vi "AlliGator Compute Lifetime Simulation Histograms.vi"(0 "tau 1":dbl[](array[numeric]), 5 "tau 2":dbl[](array[numeric]), 7 "a1":dbl[](array[numeric]), 9 "Histogram Options":T1={"Histogram Bin Size (Lifetime)"=1.0000000000000002e-10, "Histogram Bin Size (a1)"=0.1, "Histogram Upper Percentile"=100.0, "Histogram Lower Percentile"=0.0, "Histogram Fit"=FALSE}, 11 "Error In":errorcluster) -> (3 "Histograms":cluster{"Axis":dbl[], "Histogram":dbl[]}[](array[cluster]), 4 "Array Statistic (tau 1)":T2, 6 "Array Statistics (tau 2)":T2, 8 "Array Statistics (a1)":T2, 10 "Array of Scales":cluster{"X Scale":u32, "Y Scale":u32}[](array[cluster]), 13 "Plot Names":string[](array[string]), 14 "Message":string, 15 "Error Out":errorcluster)   [LabVIEW 2021, in "AlliGator Fit Method Benchmark.lvlib"]
doc: "Computes fitted parameter histograms and statistics."
uses:
  AlliGator Fit Method Benchmark.lvlib
  Arrays/Array Statistics.ctl
  AlliGator FMB Histogram Options.ctl
  Histograms/Linear Histogram Options.ctl
  Histograms/Histogram Bin Option.ctl
  Histograms/Histogram Bin Position.ctl
  5e0c3266-499e-46b2-80ef-c194e49f915b.vi
  9765538f-b151-4b8e-9b71-29b00fbc2fe4.vi
  8faa86fc-1a47-49e1-a18e-559db2184d30.vi
  c2a6bf4c-2b36-4ed5-885f-cf0e0406484b.vi
  6ac06ea2-d37e-43e0-baed-35fadc42c3ab.vi
  6045f332-e983-43bb-9ace-d0f5cff48457.vi
  dfa1e9a8-16d4-484e-b1d6-6a58a8855e91.vi
  5e0c3266-499e-46b2-80ef-c194e49f915b.vi/1ce800e1-bcd7-4855-83e2-66cab3687e54.vi
  9765538f-b151-4b8e-9b71-29b00fbc2fe4.vi/1ce800e1-bcd7-4855-83e2-66cab3687e54.vi
  8faa86fc-1a47-49e1-a18e-559db2184d30.vi/1ce800e1-bcd7-4855-83e2-66cab3687e54.vi
  c2a6bf4c-2b36-4ed5-885f-cf0e0406484b.vi/b1828c6e-eb0a-43e9-a724-8b596c52e435.vi
  c2a6bf4c-2b36-4ed5-885f-cf0e0406484b.vi/7a6138ed-c001-4311-b538-9ba42ae7c7b1.vi
  c2a6bf4c-2b36-4ed5-885f-cf0e0406484b.vi/52c6b4fa-501b-4af0-803b-8bab516ca5d3.vi
  c2a6bf4c-2b36-4ed5-885f-cf0e0406484b.vi/d7237e10-35ab-4bcb-a0c6-4883c3f4c990.vi
  c2a6bf4c-2b36-4ed5-885f-cf0e0406484b.vi/5fb5dd96-3b97-4592-ba56-58181c8e7105.vi
  c2a6bf4c-2b36-4ed5-885f-cf0e0406484b.vi/8e13a849-a393-4484-9968-4af7b25c38d7.vi
  6ac06ea2-d37e-43e0-baed-35fadc42c3ab.vi/b1828c6e-eb0a-43e9-a724-8b596c52e435.vi
  6ac06ea2-d37e-43e0-baed-35fadc42c3ab.vi/7a6138ed-c001-4311-b538-9ba42ae7c7b1.vi
  6ac06ea2-d37e-43e0-baed-35fadc42c3ab.vi/52c6b4fa-501b-4af0-803b-8bab516ca5d3.vi
  6ac06ea2-d37e-43e0-baed-35fadc42c3ab.vi/d7237e10-35ab-4bcb-a0c6-4883c3f4c990.vi
  6ac06ea2-d37e-43e0-baed-35fadc42c3ab.vi/5fb5dd96-3b97-4592-ba56-58181c8e7105.vi
  6ac06ea2-d37e-43e0-baed-35fadc42c3ab.vi/8e13a849-a393-4484-9968-4af7b25c38d7.vi
  6045f332-e983-43bb-9ace-d0f5cff48457.vi/b1828c6e-eb0a-43e9-a724-8b596c52e435.vi
  6045f332-e983-43bb-9ace-d0f5cff48457.vi/7a6138ed-c001-4311-b538-9ba42ae7c7b1.vi
  6045f332-e983-43bb-9ace-d0f5cff48457.vi/52c6b4fa-501b-4af0-803b-8bab516ca5d3.vi
  6045f332-e983-43bb-9ace-d0f5cff48457.vi/d7237e10-35ab-4bcb-a0c6-4883c3f4c990.vi
  6045f332-e983-43bb-9ace-d0f5cff48457.vi/5fb5dd96-3b97-4592-ba56-58181c8e7105.vi
  6045f332-e983-43bb-9ace-d0f5cff48457.vi/8e13a849-a393-4484-9968-4af7b25c38d7.vi
  dfa1e9a8-16d4-484e-b1d6-6a58a8855e91.vi/b1828c6e-eb0a-43e9-a724-8b596c52e435.vi
  dfa1e9a8-16d4-484e-b1d6-6a58a8855e91.vi/7a6138ed-c001-4311-b538-9ba42ae7c7b1.vi
  dfa1e9a8-16d4-484e-b1d6-6a58a8855e91.vi/52c6b4fa-501b-4af0-803b-8bab516ca5d3.vi
  dfa1e9a8-16d4-484e-b1d6-6a58a8855e91.vi/d7237e10-35ab-4bcb-a0c6-4883c3f4c990.vi
  dfa1e9a8-16d4-484e-b1d6-6a58a8855e91.vi/5fb5dd96-3b97-4592-ba56-58181c8e7105.vi
  dfa1e9a8-16d4-484e-b1d6-6a58a8855e91.vi/8e13a849-a393-4484-9968-4af7b25c38d7.vi
  Time/High Resolution Timing.vi
  <userlib>/_OpenG.lib/array/array.llb/Filter 1D Array__ogtk.vi
  <userlib>/_OpenG.lib/array/array.llb/Filter 1D Array (DBL)__ogtk.vi
  <userlib>/_OpenG.lib/array/array.llb/Delete Elements from Array__ogtk.vi
  <userlib>/_OpenG.lib/array/array.llb/Delete Elements from 1D Array (DBL)__ogtk.vi
  <vilib>/Utility/error.llb/Error Cluster From Error Code.vi
  Histograms/Histogram Window.lvlib
  Arrays/Arrays.lvlib
  Variant/Variant.lvlib
panel:
  # "see the AlliGator License on the block diagram (Ctrl+E or Window:Show Block Diagram)"
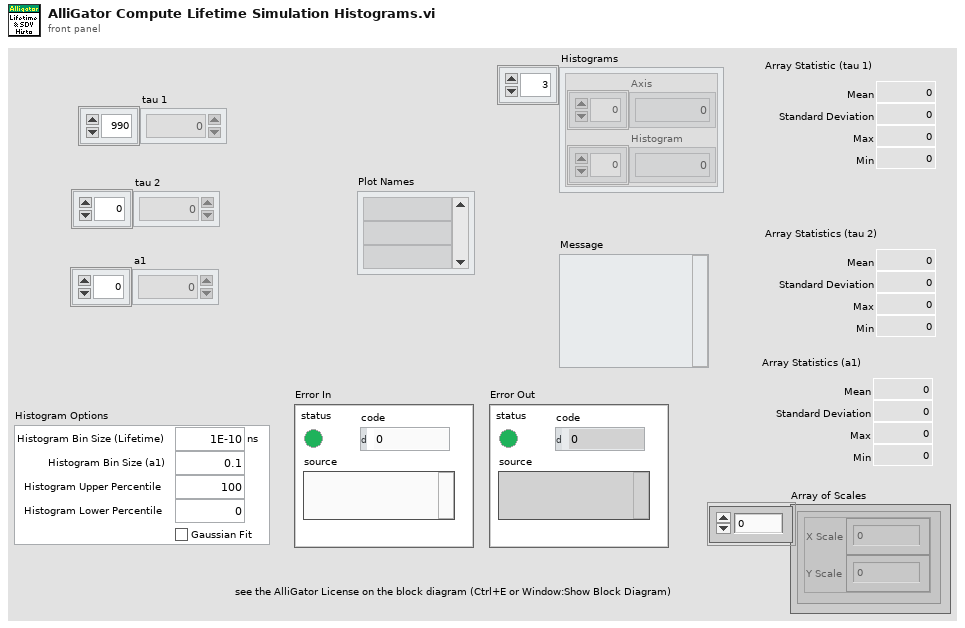
[diagram p1: front panel]
types:
  T1 = typedef "AlliGator Fit Method Benchmark.lvlib/AlliGator FMB Histogram Options.ctl" = cluster{"Histogram Bin Size (Lifetime)":dbl[unit], "Histogram Bin Size (a1)":dbl, "Histogram Upper Percentile":dbl, "Histogram Lower Percentile":dbl, "Histogram Fit":bool}
  T2 = typedef "Arrays.lvlib/Array Statistics.ctl" = cluster{"Mean":dbl, "Standard Deviation":dbl, "Max":dbl, "Min":dbl}
  T3 = typedef "Histogram Window.lvlib/Linear Histogram Options.ctl" = cluster{"Bin Size":dbl, "Bin Number":i32, "Bin Option":T4, "Min Value":dbl, "Max Value":dbl, "Filter NaN & Infinite Values":bool, "Frequency Plot":bool, "Align Bins":bool, "Bin Location":T5, "Project Outside Values":bool, "Max Histogram Size":i32}
  T4 = typedef "Histogram Window.lvlib/Histogram Bin Option.ctl" = enum32{"Bin Number", "Bin Size"}
  T5 = typedef "Histogram Window.lvlib/Histogram Bin Position.ctl" = enum16{"Left", "Center", "Right"}
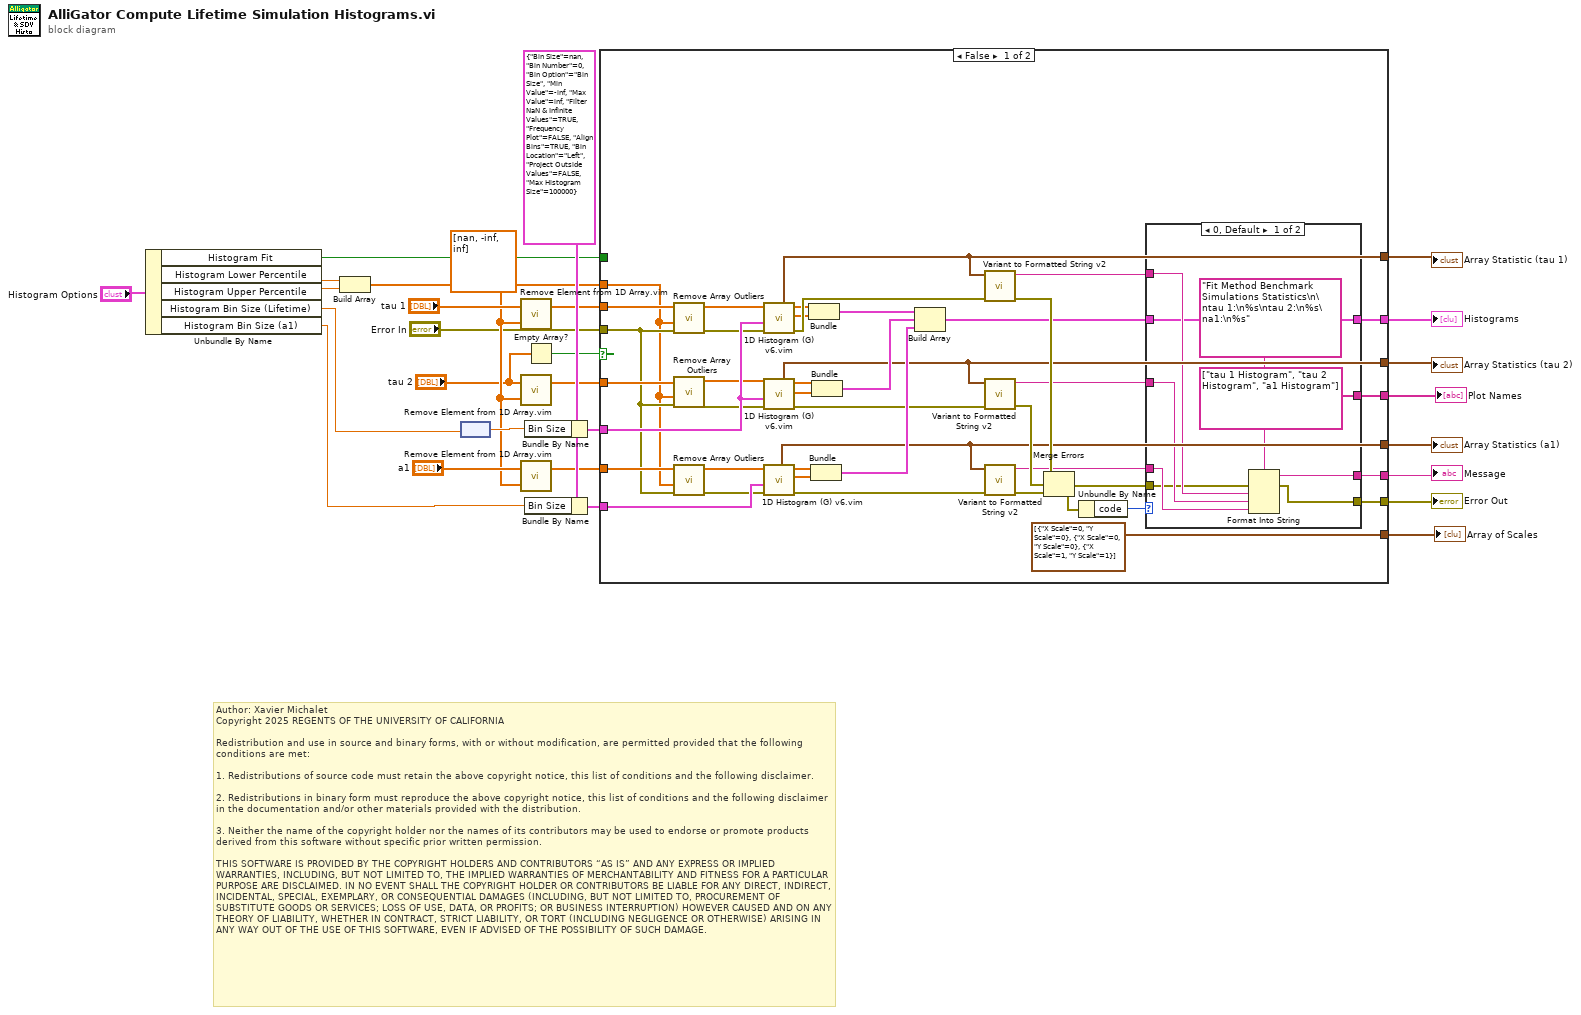
[diagram p0: block diagram]
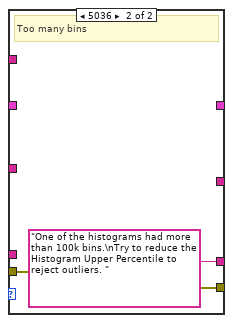
[diagram p2: hidden frame]
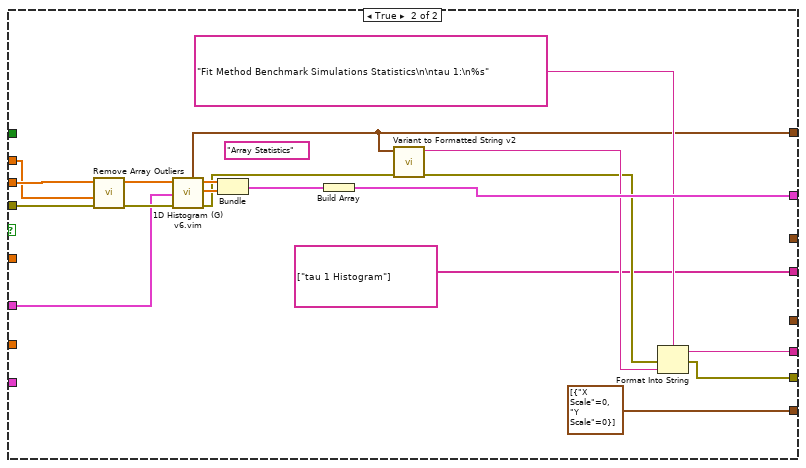
[diagram p3: hidden frame]
diagram:
  w21 = dbl[] [nan, -inf, inf] ("Element(s) to Remove")
  w27 = T3 {"Bin Size"=nan, "Bin Number"=0, "Bin Option"=enum."Bin Size", "Min Value"=-inf, "Max Value"=inf, "Filter NaN & Infinite Values"=TRUE, "Frequency Plot"=FALSE, "Align Bins"=TRUE, "Bin Location"=enum."Left", "Project Outside Values"=FALSE, "Max Histogram Size"=100000} ("Histogram Options")
  # "Author: Xavier Michalet\nCopyright 2025 REGENTS OF THE UNIVERSITY OF CALIFORNIA\n\nRedistribution and use in source and binary forms, with or without modification, are permitted provided that the following conditions are met:\n\n1. Redistributions of source code must retain the above copyright notice, this list of conditions and the following disclaimer.\n\n2. Redistributions in binary form must reproduce the above copyright notice, this list of conditions and the following disclaimer in the documentation and/or other materials provided with the distribution.\n\n3. Neither the name of the copyright holder nor the names of its contributors may be used to endorse or promote products derived from this software without specific prior written permission.\n\nTHIS SOFTWARE IS PROVIDED BY THE COPYRIGHT HOLDERS AND CONTRIBUTORS “AS IS” AND ANY EXPRESS OR IMPLIED WARRANTIES, INCLUDING, BUT NOT LIMITED TO, THE IMPLIED WARRANTIES OF MERCHANTABILITY AND FITNESS FOR A PARTICULAR PURPOSE ARE DISCLAIMED. IN NO EVENT SHALL THE COPYRIGHT HOLDER OR CONTRIBUTORS BE LIABLE FOR ANY DIRECT, INDIRECT, INCIDENTAL, SPECIAL, EXEMPLARY, OR CONSEQUENTIAL DAMAGES (INCLUDING, BUT NOT LIMITED TO, PROCUREMENT OF SUBSTITUTE GOODS OR SERVICES; LOSS OF USE, DATA, OR PROFITS; OR BUSINESS INTERRUPTION) HOWEVER CAUSED AND ON ANY THEORY OF LIABILITY, WHETHER IN CONTRACT, STRICT LIABILITY, OR TORT (INCLUDING NEGLIGENCE OR OTHERWISE) ARISING IN ANY WAY OUT OF THE USE OF THIS SOFTWARE, EVEN IF ADVISED OF THE POSSIBILITY OF SUCH DAMAGE."
  n1 = Unbundle By Name("Histogram Options") -> ("Histogram Fit"=w1:bool, "Histogram Lower Percentile"=w4:dbl, "Histogram Upper Percentile"=w3:dbl, "Histogram Bin Size (Lifetime)"=w6:dbl[unit], "Histogram Bin Size (a1)"=w5:dbl)
  n2 = Build Array(w4, w3) -> (w2:dbl[])
  n3 = node(w6) -> (w24:dbl)
  n4 = call "Remove Element from 1D Array.vim"("Element(s) to Remove"=w21, "Input Array"="tau 1") -> ("Output Array"=w15:dbl[])  [unwired: 1 out]
  n5 = call "Remove Element from 1D Array.vim"("Element(s) to Remove"=w21, "Input Array"="tau 2") -> ("Output Array"=w14:dbl[])  [unwired: 1 out]
  n6 = call "Remove Element from 1D Array.vim"("Element(s) to Remove"=w21, "Input Array"="a1") -> ("Output Array"=w13:dbl[])  [unwired: 1 out]
  n7 = Bundle By Name(cluster=w27, "Bin Size"=w24) -> (w22:T3)
  n8 = Bundle By Name(cluster=w27, "Bin Size"=w5) -> (w28:T3)
  n9 = Empty Array?(array="tau 2") -> (empty?=w10:bool)
  n10 = case shown="False" w10 {
    tunnel: w28 -> [w70 _]
    tunnel: [w39 w100] -> w23
    tunnel: w22 -> [w66 w86]
    tunnel: [w65 w96] -> w20
    tunnel: [w64 w95] -> w19
    tunnel: [w36 _] -> w18
    tunnel: [w37 _] -> w17
    tunnel: [w38 w92] -> w16
    tunnel: w15 -> [w53 w85]
    tunnel: w14 -> [w51 _]
    tunnel: w13 -> [w48 _]
    tunnel: "Error In" -> [w45 w89]
    tunnel: w2 -> [w44 w84]
    tunnel: [w43 string[] ["tau 1 Histogram"] ("Plot Names")] -> w9
    tunnel: [cluster{"X Scale":u32, "Y Scale":u32}[] [{"X Scale"=0, "Y Scale"=0}, {"X Scale"=0, "Y Scale"=0}, {"X Scale"=1, "Y Scale"=1}] ("Array of Scales") cluster{"X Scale":u32, "Y Scale":u32}[] [{"X Scale"=0, "Y Scale"=0}] ("Array of Scales")] -> w8
    tunnel: w1 -> [_ _]
    frame False {
      n11 = call "Remove Array Outliers.vi"("Error In"=w45, "Upper & Lower Percentile (100, 0)"=w44, "Array in"=w53) -> ("Error Out"=w52:errorcluster, "Array out"=w54:dbl[])  [unwired: 6 in, 1 out]
      n12 = call "Remove Array Outliers.vi"("Error In"=w45, "Upper & Lower Percentile (100, 0)"=w44, "Array in"=w51) -> ("Error Out"=w49:errorcluster, "Array out"=w50:dbl[])  [unwired: 6 in, 1 out]
      n13 = call "Remove Array Outliers.vi"("Error In"=w45, "Upper & Lower Percentile (100, 0)"=w44, "Array in"=w48) -> ("Error Out"=w46:errorcluster, "Array out"=w47:dbl[])  [unwired: 6 in, 1 out]
      n14 = call "1D Histogram (G) v6.vim"("Error In"=w52, "Histogram Options"=w66, "Array"=w54) -> ("Error Out"=w63:errorcluster, "Histogram"=w30:dbl[], "Axis"=w29:dbl[], "Array Statistics"=w38:T2)  [unwired: 2 in, 3 out]
      n15 = call "1D Histogram (G) v6.vim"("Error In"=w49, "Histogram Options"=w66, "Array"=w50) -> ("Error Out"=w62:errorcluster, "Histogram"=w32:dbl[], "Axis"=w31:dbl[], "Array Statistics"=w37:T2)  [unwired: 2 in, 3 out]
      n16 = call "1D Histogram (G) v6.vim"("Error In"=w46, "Histogram Options"=w70, "Array"=w47) -> ("Error Out"=w61:errorcluster, "Histogram"=w34:dbl[], "Axis"=w33:dbl[], "Array Statistics"=w36:T2)  [unwired: 2 in, 3 out]
      n17 = Bundle("Axis"=w29, "Histogram"=w30) -> (w67:cluster{"Axis":dbl[], "Histogram":dbl[]})  [unwired: 1 in]
      n18 = Bundle("Axis"=w33, "Histogram"=w34) -> (w69:cluster{"Axis":dbl[], "Histogram":dbl[]})  [unwired: 1 in]
      n19 = Bundle("Axis"=w31, "Histogram"=w32) -> (w68:cluster{"Axis":dbl[], "Histogram":dbl[]})  [unwired: 1 in]
      n20 = Build Array(w67, w68, w69) -> (w40:cluster{"Axis":dbl[], "Histogram":dbl[]}[])
      n21 = call "Variant to Formatted String v2.vi"("error in (no error)"=w63, "Anything"=w38) -> ("error out"=w60:errorcluster, "String"=w57:string)  [unwired: 8 in]
      n22 = call "Variant to Formatted String v2.vi"("error in (no error)"=w62, "Anything"=w37) -> ("error out"=w59:errorcluster, "String"=w56:string)  [unwired: 8 in]
      n23 = call "Variant to Formatted String v2.vi"("error in (no error)"=w61, "Anything"=w36) -> ("error out"=w58:errorcluster, "String"=w55:string)  [unwired: 8 in]
      n24 = Merge Errors(w60, w59, w58) -> (w42:errorcluster)
      n25 = Unbundle By Name(w42) -> ("code"=w41:i32)
      n26 = case shown="0, Default" w41 {
        tunnel: [w79 "One of the histograms had more than 100k bins.\nTry to reduce the Histogram Upper Percentile to reject outliers. "] -> w65
        tunnel: [w78 w81] -> w64
        tunnel: w57 -> [w77 _]
        tunnel: w56 -> [w76 _]
        tunnel: w55 -> [w75 _]
        tunnel: [string[] ["tau 1 Histogram", "tau 2 Histogram", "a1 Histogram"] ("Plot Names") _] -> w43
        tunnel: w42 -> [w73 w81]
        tunnel: w40 -> [w72 _]
        tunnel: [w72 _] -> w39
        frame 0, Default {
          n27 = Format Into String(format string="Fit Method Benchmark Simulations Statistics\n\ntau 1:\n%s\ntau 2:\n%s\na1:\n%s", error in=w73, w77, w76, w75) -> (resulting string=w79:string, error out=w78:errorcluster)  [unwired: 1 in]
        }
        frame 5036 {
          # "Too many bins"
        }
      }
    }
    frame True {
      (unwired) "Array Statistics" ("Label")
      n28 = call "Remove Array Outliers.vi"("Error In"=w89, "Upper & Lower Percentile (100, 0)"=w84, "Array in"=w85) -> ("Error Out"=w90:errorcluster, "Array out"=w91:dbl[])  [unwired: 6 in, 1 out]
      n29 = call "1D Histogram (G) v6.vim"("Error In"=w90, "Histogram Options"=w86, "Array"=w91) -> ("Error Out"=w94:errorcluster, "Histogram"=w98:dbl[], "Axis"=w97:dbl[], "Array Statistics"=w92:T2)  [unwired: 2 in, 3 out]
      n30 = Bundle("Axis"=w97, "Histogram"=w98) -> (w99:cluster{"Axis":dbl[], "Histogram":dbl[]})  [unwired: 1 in]
      n31 = Build Array(w99) -> (w100:cluster{"Axis":dbl[], "Histogram":dbl[]}[])
      n32 = call "Variant to Formatted String v2.vi"("error in (no error)"=w94, "Anything"=w92) -> ("error out"=w87:errorcluster, "String"=w88:string)  [unwired: 8 in]
      n33 = Format Into String(format string="Fit Method Benchmark Simulations Statistics\n\ntau 1:\n%s", error in=w87, w88) -> (resulting string=w96:string, error out=w95:errorcluster)  [unwired: 1 in]
    }
  }
  "Histograms" <- w23
  "Array Statistics (tau 2)" <- w17
  "Array Statistic (tau 1)" <- w16
  "Array Statistics (a1)" <- w18
  "Error Out" <- w19
  "Message" <- w20
  "Plot Names" <- w9
  "Array of Scales" <- w8
